vi "Report.vi"(8 "error in (no error)":errorcluster, 9 "Received":path, 10 "Approved":path, 11 "Beyond Compare in":refnum<class "Beyond Compare.lvclass">) -> (0 "error out":errorcluster, 3 "Beyond Compare out":refnum<class "Beyond Compare.lvclass">)   [LabVIEW 2020, in "Approval Tests.lvlib" / "Beyond Compare.lvclass"]
uses:
  Beyond Compare.lvclass
  Beyond Compare.lvclass/Beyond Compare.ctl
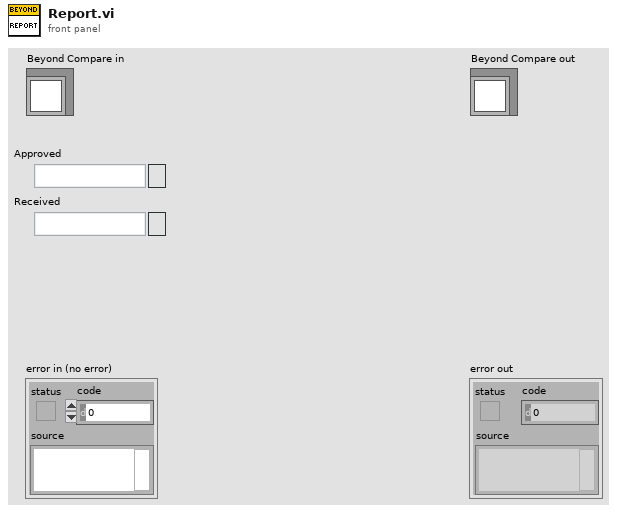
[diagram p1: front panel]
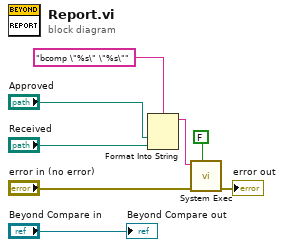
[diagram p0: block diagram]
diagram:
  n1 = Format Into String(format string="bcomp \"%s\" \"%s\"", "Approved", "Received") -> (resulting string=w2:string)  [unwired: 2 in, 1 out]
  n2 = call <vilib>:"System Exec.vi"("wait until completion? (T)"=FALSE, "error in (no error)"="error in (no error)", "command line"=w2) -> ("error out"=→"error out":errorcluster)  [unwired: 5 in, 3 out]
  "Beyond Compare out" <- "Beyond Compare in"
